vi "ClsSetOutputSignalIDs.vi"(8 "error in (no error)":errorcluster, 10 "Signal IDs array":i32[](array[numeric]), 11 "Connection In":u32) -> (0 "error out":errorcluster, 3 "Connection Out":u32)   [LabVIEW 2015]
doc: "Set Output Signal IDs:\n\nUse this function for selecting signal IDs for output. Please refer to the device manual for how signal IDs are defined in your device. Signal IDs smaller than 64 are used for CHRocodile 1 devices and Signal IDs greater or equal to 64 are used for CHRocodile 2 and multiple channel devices.\n\nConnection In[Input]: the connection handle which is initially created by Open Connection subVI.\n\nSignal IDs array[Input]: The one dimensional signal IDs array whose dimension should be no more than 32. Note: do not combine signal IDs < 64 with signal IDs >= 64.\n\nConnection Out[Output]: the connection handle output which could be used for next subVI refering to the same connection."
uses:
  dependent dlls/CHRocodileDLL.dll
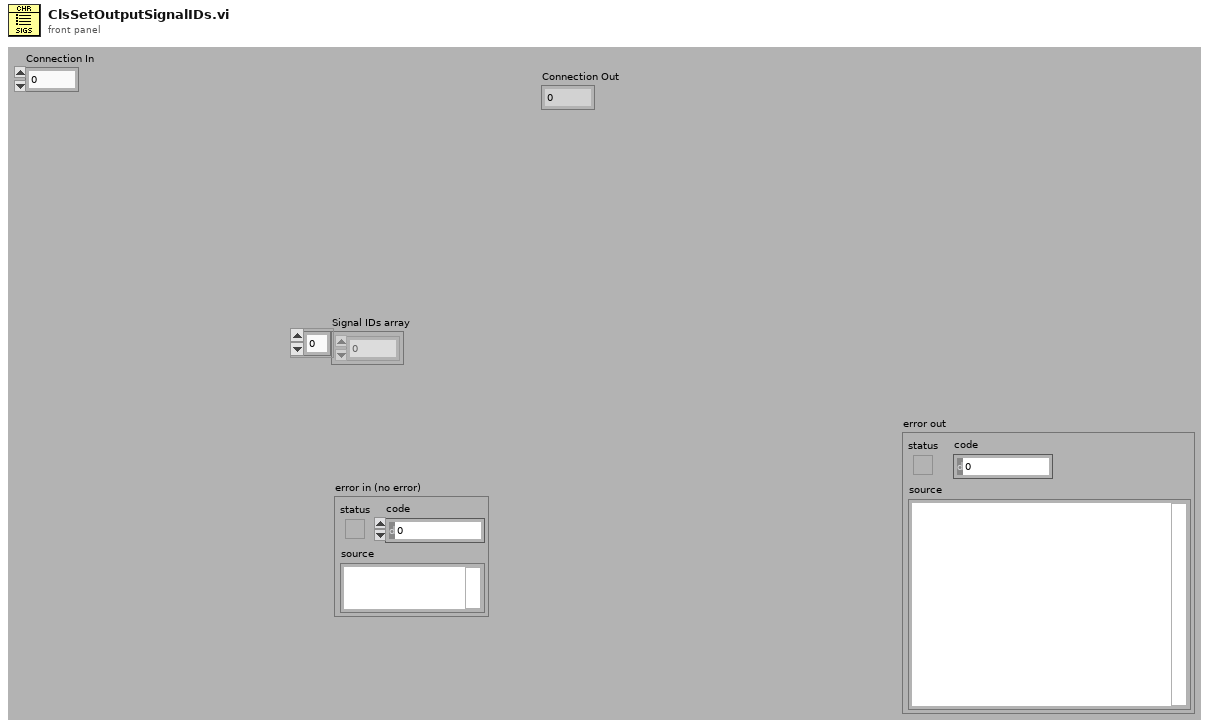
[diagram p1: front panel]
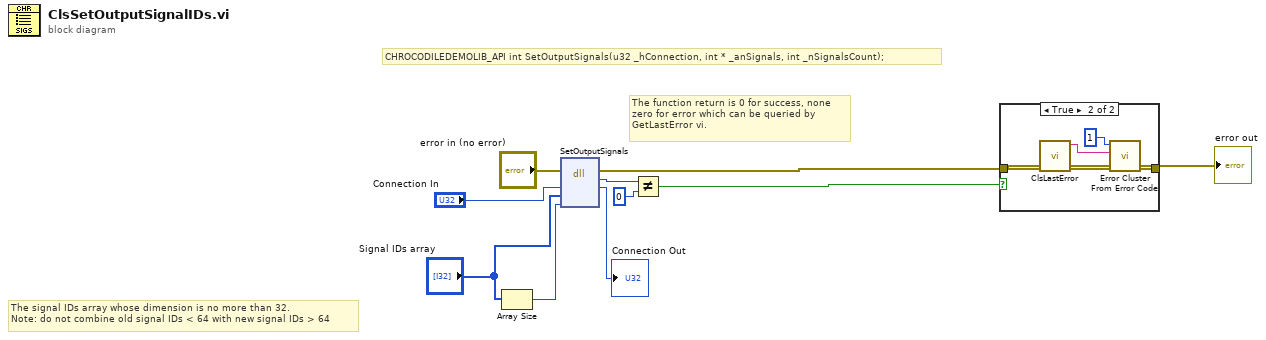
[diagram p0: block diagram]
diagram:
  # "The signal IDs array whose dimension is no more than 32.\nNote: do not combine old signal IDs < 64 with new signal IDs > 64"
  # "The function return is 0 for success, none\nzero for error which can be queried by\nGetLastError vi."
  # "CHROCODILEDEMOLIB_API int SetOutputSignals(u32 _hConnection, int * _anSignals, int _nSignalsCount);"
  n1 = Array Size(array="Signal IDs array") -> (size(s)=w2:i32)
  n2 = dll-call lib="W:/Drop Impact Teststand/dependent dlls/CHRocodileDLL.*" fn="SetOutputSignals"(error in="error in (no error)", "_hConnection"="Connection In", "_anSignals"="Signal IDs array", "_nSignalsCount"=w2) -> (error out=w5:errorcluster, "return type"=w6:i32, "_hConnection"=→"Connection Out":u32)  [unwired: 4 in, 1 out]
  n3 = Not Equal?(x=w6, y=0) -> (x != y?=w7:bool)
  n4 = case shown="True" w7 {
    tunnel: [w11 w12] -> w9
    tunnel: w5 -> [w11 w13]
    frame False {
    }
    frame True {
      n5 = call "ClsLastError.vi"("error in (no error)"=w13) -> ("error out"=w14:errorcluster, "Error Message"=w15:string)  [unwired: 9 in]
      n6 = call <vilib>:"Error Cluster From Error Code.vi"("error in (no error)"=w14, "error message (\"\")"=w15, "error code (0)"=1) -> ("error out"=w12:errorcluster)  [unwired: 6 in]
    }
  }
  "error out" <- w9
